vi "Z_HSw.vi"(6 "Data":bool, 8 "error in (no error)":errorcluster, 9 "Z_Source":T2, 10 "connect":bool, 11 "Z_HSw_in":refnum<class "Z_HSw.lvclass">) -> (0 "error out":errorcluster, 3 "Z_HSw_out":refnum<class "Z_HSw.lvclass">)   [LabVIEW 2019, in "Z_HSw.lvclass"]
uses:
  Z_HSw.lvclass
  D:/my_projects/projects/Algorithms/Labview/19/Sequence/State/State.lvclass
  Z_source.ctl
  switch_state.ctl
  Z_HSw.lvclass/Z_HSw.ctl
  Sequence/State/State.lvclass/State.ctl
  Sequence/State/State.lvclass
  Heating/ctl/Z_Hswitch_little/Y_SourceInd.ctl
  Heating/ctl/Z_Hswitch_little/Z_Hswitch_little.xctl
panel:
  out "Z1 ind":T1
  out "Z1 ind 3":u8(ring)
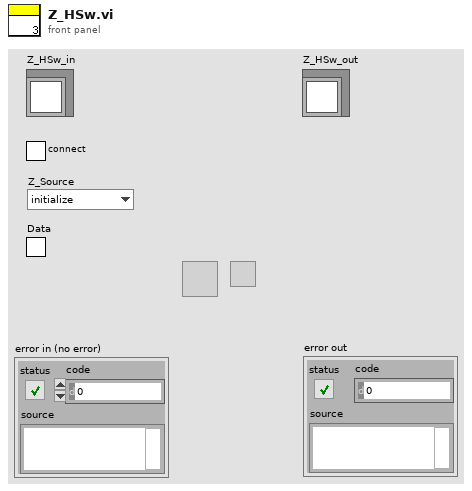
[diagram p1: front panel]
types:
  T1 = typedef "Heating.lvlib/Z_Hswitch_little.xctl/Y_SourceInd.ctl" = u8
  T2 = typedef "Z_source.ctl" = enum8{"initialize", "local disabled", "local hand", "hand", "auto", "dist"}
  T3 = typedef "switch_state.ctl" = enum16{"init", "switch off", "not off", "off", "switch on", "not on", "on"}
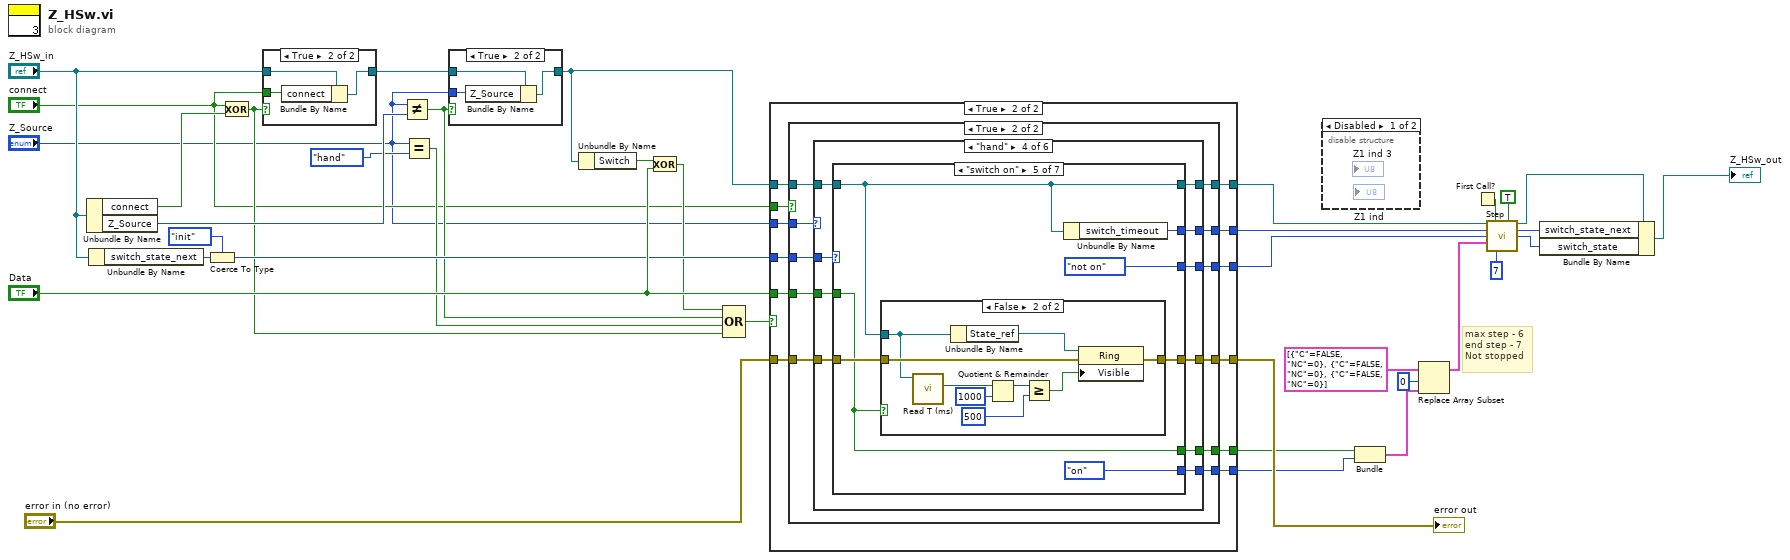
[diagram p0: block diagram]
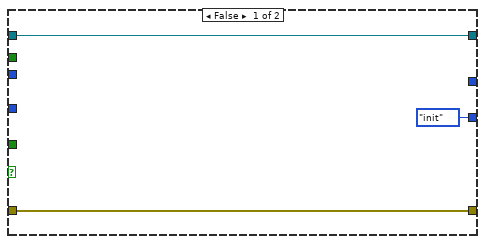
[diagram p2: hidden frame]
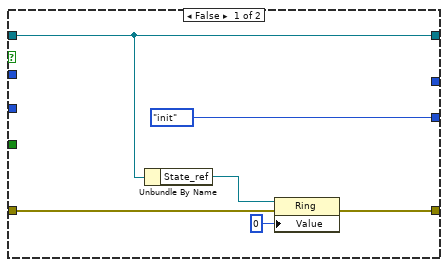
[diagram p3: hidden frame]
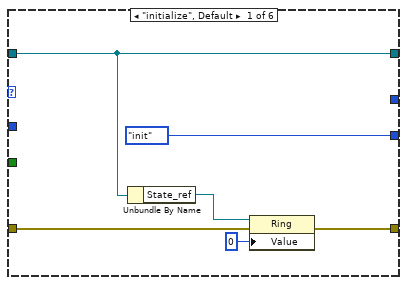
[diagram p4: hidden frame]
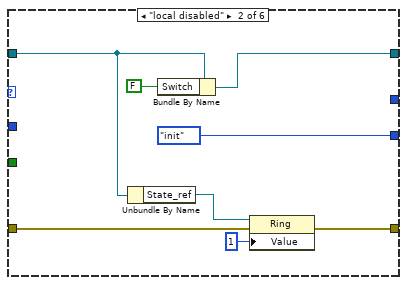
[diagram p5: hidden frame]
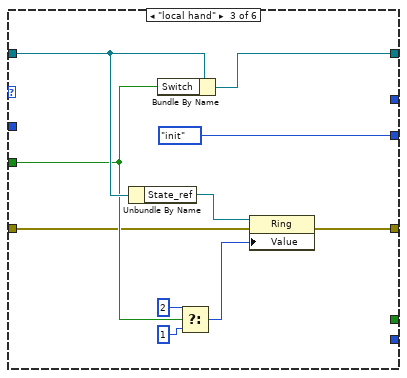
[diagram p6: hidden frame]
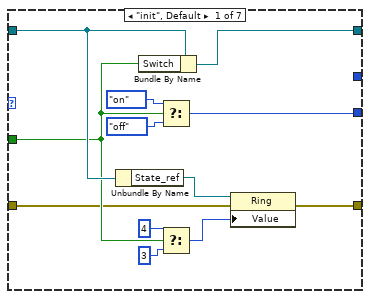
[diagram p7: hidden frame]
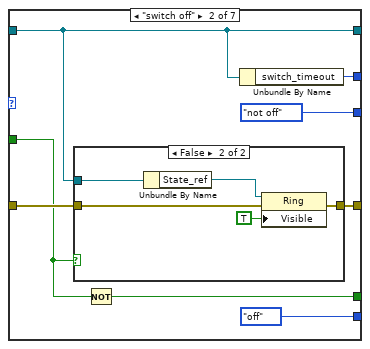
[diagram p8: hidden frame]
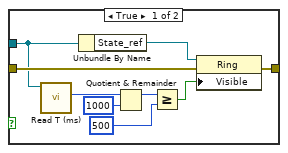
[diagram p9: hidden frame]
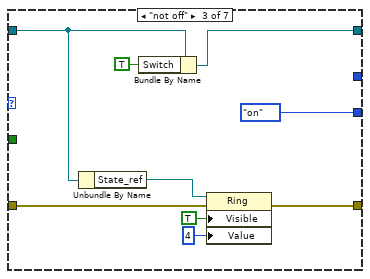
[diagram p10: hidden frame]
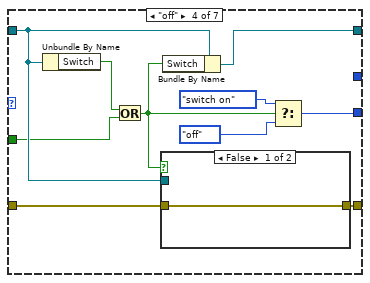
[diagram p11: hidden frame]
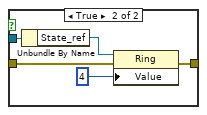
[diagram p12: hidden frame]
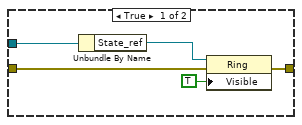
[diagram p13: hidden frame]
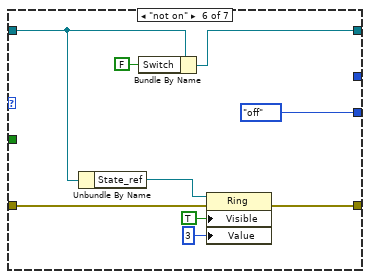
[diagram p14: hidden frame]
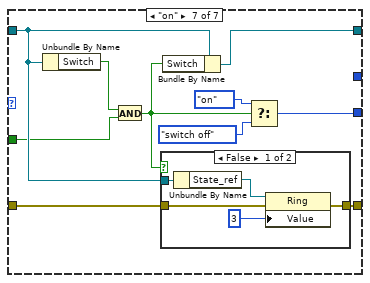
[diagram p15: hidden frame]
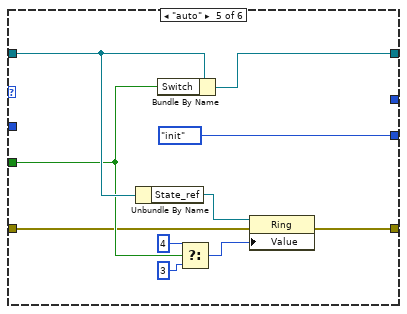
[diagram p17: hidden frame]
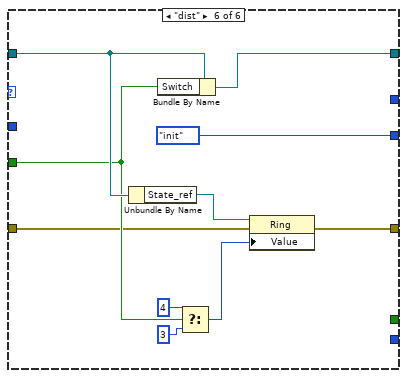
[diagram p18: hidden frame]
diagram:
  # "max step - 6\nend step - 7\nNot stopped"
  n1 = Unbundle By Name("Z_HSw_in") -> ("connect"=w15:bool, "Z_Source"=w10:T2)
  n2 = Unbundle By Name("Z_HSw_in") -> ("switch_state_next"=w22:T3)
  n3 = Coerce To Type(0:w22, 1:switch_state."init" ("switch_state")) -> (2:w9:T3)
  n4 = Exclusive Or(1:w15, 2:"connect") -> (0:w4:bool)
  n5 = case shown="True" w4 {
    tunnel: "Z_HSw_in" -> [w37 w40]
    tunnel: [w37 w39] -> w14
    tunnel: "connect" -> [_ w38]
    frame False {
    }
    frame True {
      n6 = Bundle By Name(cluster=w40, "connect"=w38) -> (w39:refnum<class "Z_HSw.lvclass">)
    }
  }
  n7 = Not Equal?(x="Z_Source", y=w10) -> (x != y?=w7:bool)
  n8 = Equal?(x="Z_Source", y=Z_source."hand" ("Z_Source")) -> (x = y?=w6:bool)
  n9 = case shown="True" w7 {
    tunnel: w14 -> [w41 w44]
    tunnel: [w41 w43] -> w13
    tunnel: "Z_Source" -> [_ w42]
    frame False {
    }
    frame True {
      n10 = Bundle By Name(cluster=w44, "Z_Source"=w42) -> (w43:refnum<class "Z_HSw.lvclass">)
    }
  }
  n11 = Unbundle By Name(w13) -> ("Switch"=w12:bool)
  n12 = Exclusive Or(1:"Data", 2:w12) -> (0:w8:bool)
  n13 = Compound Arithmetic op=OR(w8, w7, w6, w4) -> (w3:bool)
  n14 = case shown="True" w3 {
    tunnel: [switch_state."init" ("switch_state") w59] -> w25
    tunnel: "error in (no error)" -> [w45 w58]
    tunnel: [w45 w57] -> w23
    tunnel: [w47 w56] -> w21
    tunnel: [_ w55] -> w20
    tunnel: [_ w54] -> w19
    tunnel: [_ w53] -> w18
    tunnel: "connect" -> [_ w52]
    tunnel: w13 -> [w47 w51]
    tunnel: "Data" -> [_ w50]
    tunnel: "Z_Source" -> [_ w49]
    tunnel: w9 -> [_ w48]
    frame False {
    }
    frame True {
      n15 = case shown="True" w52 {
        tunnel: w49 -> [_ w76]
        tunnel: [w61 w72] -> w56
        tunnel: w50 -> [_ w75]
        tunnel: [switch_state."init" ("switch_state") w74] -> w59
        tunnel: w58 -> [w60 w71]
        tunnel: w51 -> [w61 w73]
        tunnel: [w62 w70] -> w57
        tunnel: w48 -> [_ w69]
        tunnel: [_ w68] -> w55
        tunnel: [_ w67] -> w54
        tunnel: [_ w66] -> w53
        frame False {
          n16 = Unbundle By Name(w61) -> ("State_ref"=w64:refnum<vi>)
          n17 = property on="Property Node" class="Ring"(reference=w64, error in=w60, "Value"=u8 0 ("Z1_ind visu")) -> (error out=w62:errorcluster)  [unwired: 1 out]
        }
        frame True {
          n18 = case shown="\"hand\"" w76 {
            tunnel: w75 -> [_ _ w93 w108 w218 w228]
            tunnel: [switch_state."init" ("switch_state") switch_state."init" ("switch_state") switch_state."init" ("switch_state") w107 switch_state."init" ("switch_state") switch_state."init" ("switch_state")] -> w74
            tunnel: w73 -> [w79 w85 w97 w109 w222 w232]
            tunnel: [w79 w86 w98 w110 w223 w233] -> w72
            tunnel: w71 -> [w77 w83 w92 w106 w217 w227]
            tunnel: [w80 w88 w99 w105 w224 w234] -> w70
            tunnel: w69 -> [_ _ _ w104 _ _]
            tunnel: [_ _ _ w103 _ _] -> w68
            tunnel: [_ _ _ w102 _ _] -> w67
            tunnel: [_ _ _ w101 _ _] -> w66
            frame "initialize", Default {
              # "local hand"
              n19 = Unbundle By Name(w79) -> ("State_ref"=w82:refnum<vi>)
              n20 = property on="Property Node" class="Ring"(reference=w82, error in=w77, "Value"=u8 0 ("Z1_ind visu")) -> (error out=w80:errorcluster)  [unwired: 1 out]
            }
            frame "local disabled" {
              # "local hand"
              n21 = Unbundle By Name(w85) -> ("State_ref"=w90:refnum<vi>)
              n22 = Bundle By Name(cluster=w85, "Switch"=FALSE) -> (w86:refnum<class "Z_HSw.lvclass">)
              n23 = property on="Property Node" class="Ring"(reference=w90, error in=w83, "Value"=u8 1 ("Z1_ind visu")) -> (error out=w88:errorcluster)  [unwired: 1 out]
            }
            frame "local hand" {
              # "local hand"
              n24 = Unbundle By Name(w97) -> ("State_ref"=w100:refnum<vi>)
              n25 = Bundle By Name(cluster=w97, "Switch"=w93) -> (w98:refnum<class "Z_HSw.lvclass">)
              n26 = Select(t=u8 2 ("Z1_ind visu"), s=w93, f=u8 1 ("Z1_ind visu")) -> (s? t:f=w94:u8)
              n27 = property on="Property Node" class="Ring"(reference=w100, error in=w92, "Value"=w94) -> (error out=w99:errorcluster)  [unwired: 1 out]
            }
            frame "hand" {
              # "local hand"
              n28 = case shown="\"switch on\"" w104 {
                tunnel: [w113 w123 w150 w155 w171 w196 w201] -> w110
                tunnel: w109 -> [w117 w123 w149 w158 w171 w195 w204]
                tunnel: w108 -> [w116 w124 _ w156 w170 _ w202]
                tunnel: [w114 switch_state."not off" ("switch_state") switch_state."on" ("switch_state") w159 switch_state."not on" ("switch_state") switch_state."off" ("switch_state") w205] -> w107
                tunnel: w106 -> [w111 w130 w153 w161 w176 w199 w207]
                tunnel: [w115 w129 w152 w160 w175 w198 w206] -> w105
                tunnel: [_ w128 _ _ w174 _ _] -> w103
                tunnel: [_ w126 _ _ w170 _ _] -> w102
                tunnel: [_ switch_state."off" ("switch_state") _ _ switch_state."on" ("switch_state") _ _] -> w101
                frame "init", Default {
                  n29 = Unbundle By Name(w117) -> ("State_ref"=w122:refnum<vi>)
                  n30 = Bundle By Name(cluster=w117, "Switch"=w116) -> (w113:refnum<class "Z_HSw.lvclass">)
                  n31 = Select(t=switch_state."on" ("switch_state"), s=w116, f=switch_state."off" ("switch_state")) -> (s? t:f=w114:T3)
                  n32 = Select(t=u8 4 ("Z1_ind visu"), s=w116, f=u8 3 ("Z1_ind visu")) -> (s? t:f=w121:u8)
                  n33 = property on="Property Node" class="Ring"(reference=w122, error in=w111, "Value"=w121) -> (error out=w115:errorcluster)  [unwired: 1 out]
                }
                frame "switch off" {
                  n34 = case shown="False" w124 {
                    tunnel: w130 -> [w137 w142]
                    tunnel: [w138 w143] -> w129
                    tunnel: w123 -> [w136 w141]
                    frame True {
                      n35 = call "Read T (ms).vi"("State in"=w136) -> ("T (ms)"=w132:u32)  [unwired: 9 in, 1 out]
                      n36 = Unbundle By Name(w136) -> ("State_ref"=w139:refnum<vi>)
                      n37 = Quotient & Remainder(x=w132, y=u32 1000) -> (x-y*floor(x/y)=w135:u32)  [unwired: 1 out]
                      n38 = Greater Or Equal?(x=w135, y=u32 500) -> (x >= y?=w131:bool)
                      n39 = property on="Property Node" class="Ring"(reference=w139, error in=w137, "Visible"=w131) -> (error out=w138:errorcluster)  [unwired: 1 out]
                    }
                    frame False {
                      n40 = Unbundle By Name(w141) -> ("State_ref"=w144:refnum<vi>)
                      n41 = property on="Property Node" class="Ring"(reference=w144, error in=w142, "Visible"=TRUE) -> (error out=w143:errorcluster)  [unwired: 1 out]
                    }
                  }
                  n42 = Not(x=w124) -> (.not. x?=w126:bool)
                  n43 = Unbundle By Name(w123) -> ("switch_timeout"=w128:u32)
                }
                frame "not off" {
                  n44 = Unbundle By Name(w149) -> ("State_ref"=w147:refnum<vi>)
                  n45 = Bundle By Name(cluster=w149, "Switch"=TRUE) -> (w150:refnum<class "Z_HSw.lvclass">)
                  n46 = property on="Property Node" class="Ring"(reference=w147, error in=w153, "Visible"=TRUE, "Value"=u8 4 ("Z1_ind visu")) -> (error out=w152:errorcluster)  [unwired: 1 out]
                }
                frame "off" {
                  n47 = Unbundle By Name(w158) -> ("Switch"=w157:bool)
                  n48 = Or(x=w157, y=w156) -> (x .or. y?=w154:bool)
                  n49 = case shown="False" w154 {
                    tunnel: w161 -> [w164 w166]
                    tunnel: [w164 w168] -> w160
                    tunnel: w158 -> [_ w167]
                    frame False {
                    }
                    frame True {
                      n50 = Unbundle By Name(w167) -> ("State_ref"=w169:refnum<vi>)
                      n51 = property on="Property Node" class="Ring"(reference=w169, error in=w166, "Value"=u8 4 ("Z1_ind visu")) -> (error out=w168:errorcluster)  [unwired: 1 out]
                    }
                  }
                  n52 = Bundle By Name(cluster=w158, "Switch"=w154) -> (w155:refnum<class "Z_HSw.lvclass">)
                  n53 = Select(t=switch_state."switch on" ("switch_state"), s=w154, f=switch_state."off" ("switch_state")) -> (s? t:f=w159:T3)
                }
                frame "switch on" {
                  n54 = case shown="False" w170 {
                    tunnel: w176 -> [w179 w188]
                    tunnel: [w180 w189] -> w175
                    tunnel: w171 -> [w178 w187]
                    frame True {
                      n55 = Unbundle By Name(w178) -> ("State_ref"=w181:refnum<vi>)
                      n56 = property on="Property Node" class="Ring"(reference=w181, error in=w179, "Visible"=TRUE) -> (error out=w180:errorcluster)  [unwired: 1 out]
                    }
                    frame False {
                      n57 = call "Read T (ms).vi"("State in"=w187) -> ("T (ms)"=w183:u32)  [unwired: 9 in, 1 out]
                      n58 = Unbundle By Name(w187) -> ("State_ref"=w190:refnum<vi>)
                      n59 = Quotient & Remainder(x=w183, y=u32 1000) -> (x-y*floor(x/y)=w186:u32)  [unwired: 1 out]
                      n60 = Greater Or Equal?(x=w186, y=u32 500) -> (x >= y?=w182:bool)
                      n61 = property on="Property Node" class="Ring"(reference=w190, error in=w188, "Visible"=w182) -> (error out=w189:errorcluster)  [unwired: 1 out]
                    }
                  }
                  n62 = Unbundle By Name(w171) -> ("switch_timeout"=w174:u32)
                }
                frame "not on" {
                  n63 = Unbundle By Name(w195) -> ("State_ref"=w193:refnum<vi>)
                  n64 = Bundle By Name(cluster=w195, "Switch"=FALSE) -> (w196:refnum<class "Z_HSw.lvclass">)
                  n65 = property on="Property Node" class="Ring"(reference=w193, error in=w199, "Visible"=TRUE, "Value"=u8 3 ("Z1_ind visu")) -> (error out=w198:errorcluster)  [unwired: 1 out]
                }
                frame "on" {
                  n66 = Unbundle By Name(w204) -> ("Switch"=w203:bool)
                  n67 = And(x=w203, y=w202) -> (x .and. y?=w200:bool)
                  n68 = case shown="False" w200 {
                    tunnel: w207 -> [w211 w215]
                    tunnel: [w213 w215] -> w206
                    tunnel: w204 -> [w212 _]
                    frame False {
                      n69 = Unbundle By Name(w212) -> ("State_ref"=w214:refnum<vi>)
                      n70 = property on="Property Node" class="Ring"(reference=w214, error in=w211, "Value"=u8 3 ("Z1_ind visu")) -> (error out=w213:errorcluster)  [unwired: 1 out]
                    }
                    frame True {
                    }
                  }
                  n71 = Bundle By Name(cluster=w204, "Switch"=w200) -> (w201:refnum<class "Z_HSw.lvclass">)
                  n72 = Select(t=switch_state."on" ("switch_state"), s=w200, f=switch_state."switch off" ("switch_state")) -> (s? t:f=w205:T3)
                }
              }
            }
            frame "auto" {
              # "local hand"
              n73 = Unbundle By Name(w222) -> ("State_ref"=w225:refnum<vi>)
              n74 = Bundle By Name(cluster=w222, "Switch"=w218) -> (w223:refnum<class "Z_HSw.lvclass">)
              n75 = Select(t=u8 4 ("Z1_ind visu"), s=w218, f=u8 3 ("Z1_ind visu")) -> (s? t:f=w219:u8)
              n76 = property on="Property Node" class="Ring"(reference=w225, error in=w217, "Value"=w219) -> (error out=w224:errorcluster)  [unwired: 1 out]
            }
            frame "dist" {
              # "local hand"
              n77 = Unbundle By Name(w232) -> ("State_ref"=w235:refnum<vi>)
              n78 = Bundle By Name(cluster=w232, "Switch"=w228) -> (w233:refnum<class "Z_HSw.lvclass">)
              n79 = Select(t=u8 4 ("Z1_ind visu"), s=w228, f=u8 3 ("Z1_ind visu")) -> (s? t:f=w229:u8)
              n80 = property on="Property Node" class="Ring"(reference=w235, error in=w227, "Value"=w229) -> (error out=w234:errorcluster)  [unwired: 1 out]
            }
          }
        }
      }
    }
  }
  "error out" <- w23
  n81 = disable-structure shown="Disabled" {
    frame Disabled {
    }
    frame Enabled {
    }
  }
  n82 = Bundle("Data"=w19, "switch_state"=w18) -> (w27:cluster{"Data":bool, "switch_state":T3})  [unwired: 1 in]
  n83 = Replace Array Subset(array=cluster{"C":bool, "NC":u32}[] [{"C"=FALSE, "NC"=0}, {"C"=FALSE, "NC"=0}, {"C"=FALSE, "NC"=0}] ("appended array"), new element=w27, index=0) -> (w26:cluster{"C":bool, "NC":u32}[])
  n84 = First Call?() -> (First Call?: T/F=w36:bool)
  n85 = call "Step.vi"("State in"=w21, "Reset"=w36, "Start in"=TRUE ("Start"), "t"=w20, "Nt"=w25, "C_table"=w26, "N end step"=u32 7) -> ("State out"=w31:refnum<class "Z_HSw.lvclass">, "N next"=w34:u32, "N curr"=w35:u32)  [unwired: 5 in, 1 out]
  n86 = Bundle By Name(cluster=w31, "switch_state_next"=w34, "switch_state"=w35) -> (→"Z_HSw_out":refnum<class "Z_HSw.lvclass">)
